vi "GetInstalledPythonVersions.vi"(8 "Error In":errorcluster) -> (0 "Error Out":errorcluster, 1 "Python Versions[]":T1[](array[typedef]), 2 "python.exe --version":string[](array[string]), 3 "found python.exe":string[](array[string]))   [LabVIEW 2014]
uses:
  <userlib>/_OpenG.lib/string/string.llb/Trim Whitespace (String)__ogtk.vi
  <vilib>/regexp/Match Regular Expression.xnode
  <vilib>/AppBuilder/AB_API_Simple/Build Specification Version.ctl
  <vilib>/AppBuilder/AB_API_Simple/NI_App_Builder_API.lvlib
panel:
  out "standard output":string
  out "standard error":string
  # "Get the version of the installed Python distributions\n\nNote: the path must be added to the system variables, \notherwise LabVIEW wont find any python.exe at all"
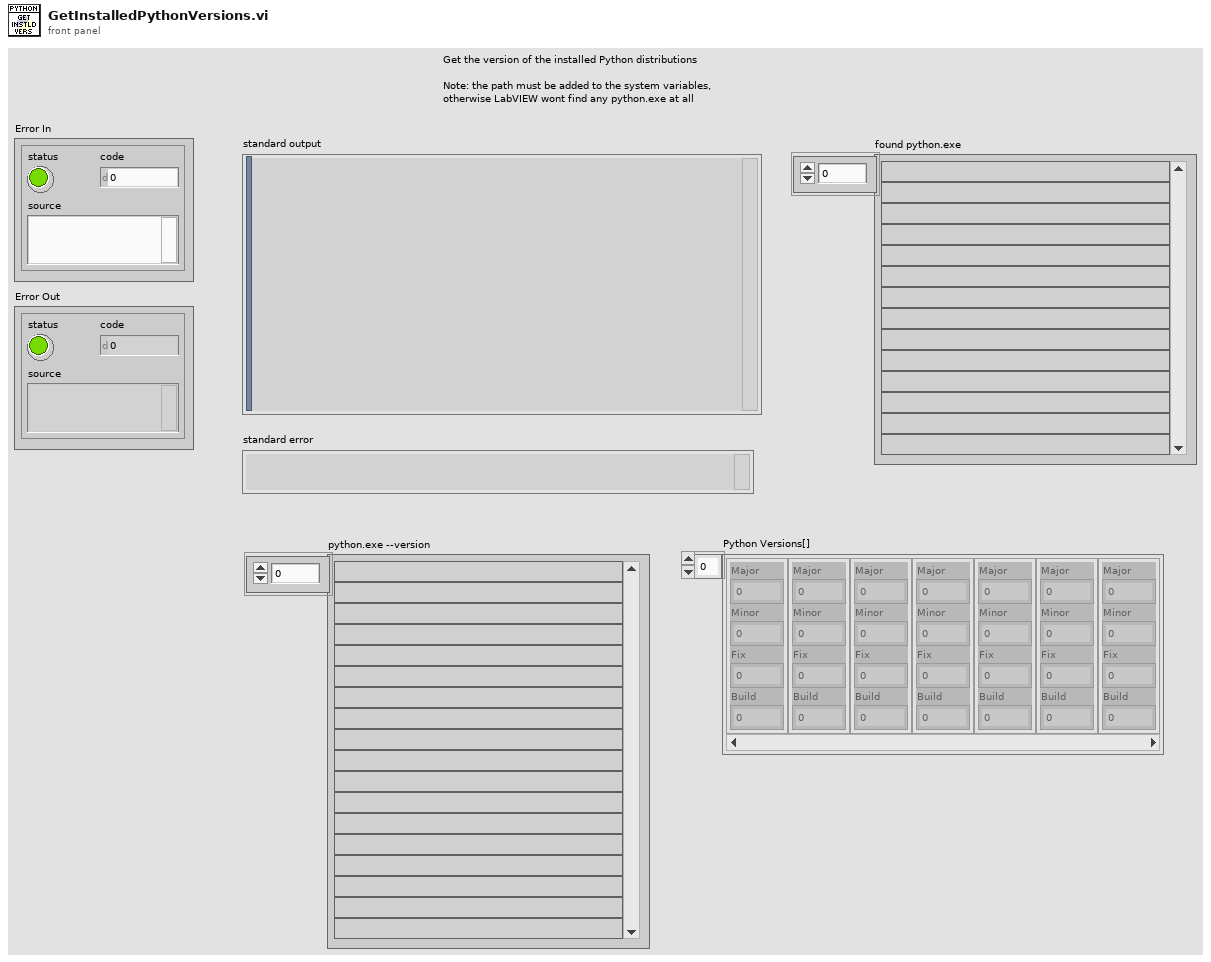
[diagram p1: front panel]
types:
  T1 = typedef "NI_App_Builder_API.lvlib/Build Specification Version.ctl" = cluster{"Major":u16, "Minor":u16, "Fix":u16, "Build":u16}
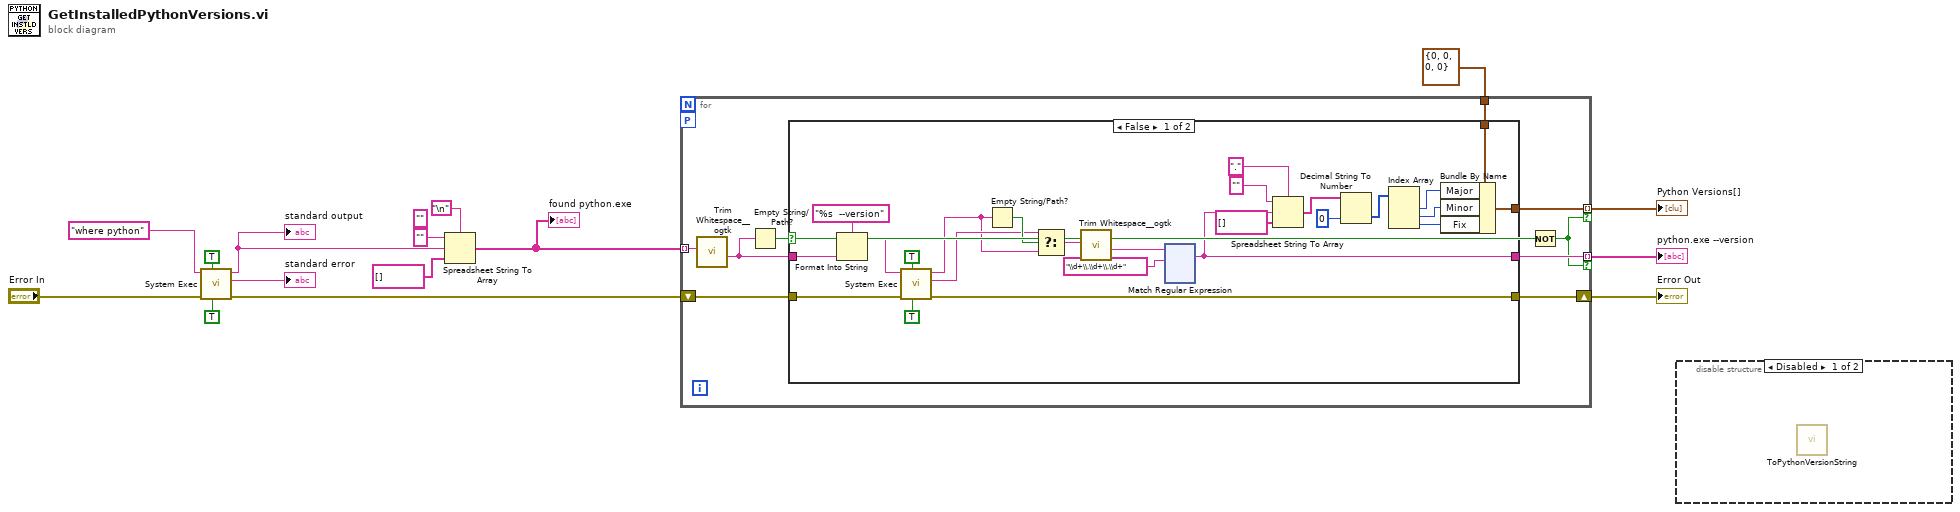
[diagram p0: block diagram]
diagram:
  (unwired) "" ("delimiter (Tab)")
  n1 = call <vilib>:"System Exec.vi"("run minimized? (F)"=TRUE, "wait until completion? (T)"=TRUE, "error in (no error)"="Error In", "command line"="where python") -> ("error out"=w8:errorcluster, "standard error"=→"standard error":string, "standard output"=w10:string)  [unwired: 4 in, 1 out]
  "standard output" <- w10
  n2 = Spreadsheet String To Array(delimiter (Tab)="\n", format string="", spreadsheet string=w10, array type (2D Dbl)=string[] [] ("found python.exe")) -> (array=w7:string[])
  "found python.exe" <- w7
  n3 = for {
    tunnel: w7 -> [w22] mode=indexing
    tunnel: [w21] -> w3 mode=indexing if=w16
    workers-P: _ -> [_]
    shift-right: [w23] -> w6
    shift-left: w8 -> [w24]
    tunnel: T1 {"Major"=0, "Minor"=0, "Fix"=0, "Build"=0} ("Build Specification Version") -> [w18]
    tunnel: [w17] -> w1 mode=indexing if=w16
    n4 = call-poly <userlib>:"Trim Whitespace__ogtk.vi"("String in"=w22) -> ("String out"=w20:string)  [unwired: 6 in]
    n5 = Empty String/Path?(string/path=w20) -> (empty?=w19:bool)
    n6 = case shown="False" w19 {
      tunnel: w24 -> [w47 w166]
      tunnel: [w44 w166] -> w23
      tunnel: w20 -> [w43 w165]
      tunnel: [w30 w165] -> w21
      tunnel: w18 -> [w36 w164]
      tunnel: [w35 w164] -> w17
      frame False {
        n7 = Format Into String(format string="%s  --version" ("command line"), w43) -> (resulting string=w45:string)  [unwired: 2 in, 1 out]
        n8 = call <vilib>:"System Exec.vi"("run minimized? (F)"=TRUE, "wait until completion? (T)"=TRUE, "error in (no error)"=w47, "command line"=w45) -> ("error out"=w44:errorcluster, "standard error"=w41:string, "standard output"=w39:string)  [unwired: 4 in, 1 out]
        n9 = Empty String/Path?(string/path=w39) -> (empty?=w42:bool)
        n10 = Select(t=w41, s=w42, f=w39) -> (s? t:f=w40:string)
        n11 = call-poly <userlib>:"Trim Whitespace__ogtk.vi"("String in"=w40) -> ("String out"=w38:string)  [unwired: 6 in]
        n12 = xnode "Match Regular Expression"("input string"=w38, "regular expression"="\\d+\\.\\d+\\.\\d+") -> ("whole match"=w30:string)  [unwired: 4 in, 4 out]
        n13 = Spreadsheet String To Array(delimiter (Tab)=".", format string="", spreadsheet string=w30, array type (2D Dbl)=string[] [] ("found python.exe")) -> (array=w31:string[])
        n14 = Decimal String To Number(string=w31, default (0L)=u16 0 ("default (0 I32)")) -> (number=w29:u16[])  [unwired: 1 in, 1 out]
        n15 = Index Array(array=w29) -> (element #1=w28:u16, element #2=w27:u16, element #3=w26:u16)  [unwired: 3 in]
        n16 = Bundle By Name(cluster=w36, "Major"=w28, "Minor"=w27, "Fix"=w26) -> (w35:T1)
      }
      frame True {
      }
    }
    n17 = Not(x=w19) -> (.not. x?=w16:bool)
  }
  "Error Out" <- w6
  "python.exe --version" <- w3
  "Python Versions[]" <- w1
  n18 = disable-structure shown="Disabled" {
    frame Disabled {
      n19 = call "ToPythonVersionString.vi"() -> ()  [unwired: 11 in, 1 out]
    }
    frame Enabled {
    }
  }
